vi "Set Window Title.vi"(0 "Calling VI":refnum<vi>, 5 "Current DAQ Ref":refnum<vi>) -> ()   [LabVIEW 2019]
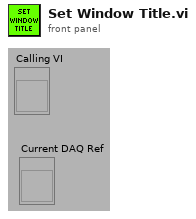
[diagram p1: front panel]
types:
  T1 = enum32{"invalid app kind", "Development System", "Run Time System", "Student Edition", "Embedded LabVIEW", "Evaluation", "Custom"}
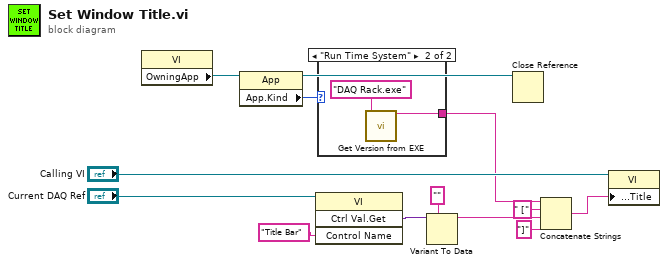
[diagram p0: block diagram]
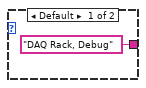
[diagram p2: hidden frame]
diagram:
  n1 = property class="VI"() -> ("OwningApp"=w4:refnum<vi>)  [unwired: 2 in, 2 out]
  n2 = property class="App"(reference=w4) -> (reference out=w1:refnum<vi>, "App.Kind"=w5:T1)  [unwired: 1 in, 1 out]
  n3 = invoke class="VI" method="Ctrl Val.Get"(reference="Current DAQ Ref", "Control Name"="Title Bar") -> ("Get Control Value Variant"=w9:variant)  [unwired: 2 in, 3 out]
  n4 = case shown="\"Run Time System\"" w5 {
    tunnel: ["DAQ Rack, Debug" ("Name and Version") w16] -> w2
    frame Default {
    }
    frame "Run Time System" {
      n5 = call "Get Version from EXE.vi"("EXE Name"="DAQ Rack.exe") -> ("Name and Version"=w16:string)  [unwired: 12 in, 2 out]
    }
  }
  n6 = Variant To Data(type="", Variant=w9) -> (data=w6:string)  [unwired: 1 in, 1 out]
  n7 = Close Reference(reference=w1) -> ()  [unwired: 1 in, 1 out]
  n8 = Concatenate Strings(w2, " [" ("string"), w6, "]" ("string")) -> (w11:string)
  n9 = property class="VI"(reference="Calling VI", "Front Panel Window:Title"=w11) -> ()  [unwired: 1 in, 2 out]
